vi "DiffDriveTrainSim_KitBotWheelSize.vi"(11 "Wheel Size":T1) -> (3 "WheelDiameter_M":dbl)   [LabVIEW 2019, in "Trajectory_Library.lvlib"]
doc: "Convience function to allow user to select kit bot wheels size from an enum selector and return the diameter in meters.\n\nInput:\n - Wheel Size -- Enumerated heel size selector\n\nOutput:\n - WheelDiameter_M -- Wheel diameter in meters."
uses:
  Trajectory_Library.lvlib
  Enum/DIFF_DRIVE_KitBot_WheelSize_ENUM.ctl
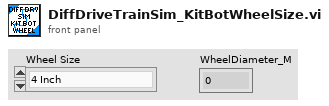
[diagram p1: front panel]
types:
  T1 = typedef "Trajectory_Library.lvlib/DIFF_DRIVE_KitBot_WheelSize_ENUM.ctl" = enum16{"4 Inch", "6 Inch", "8 Inch", "10 Inch"}
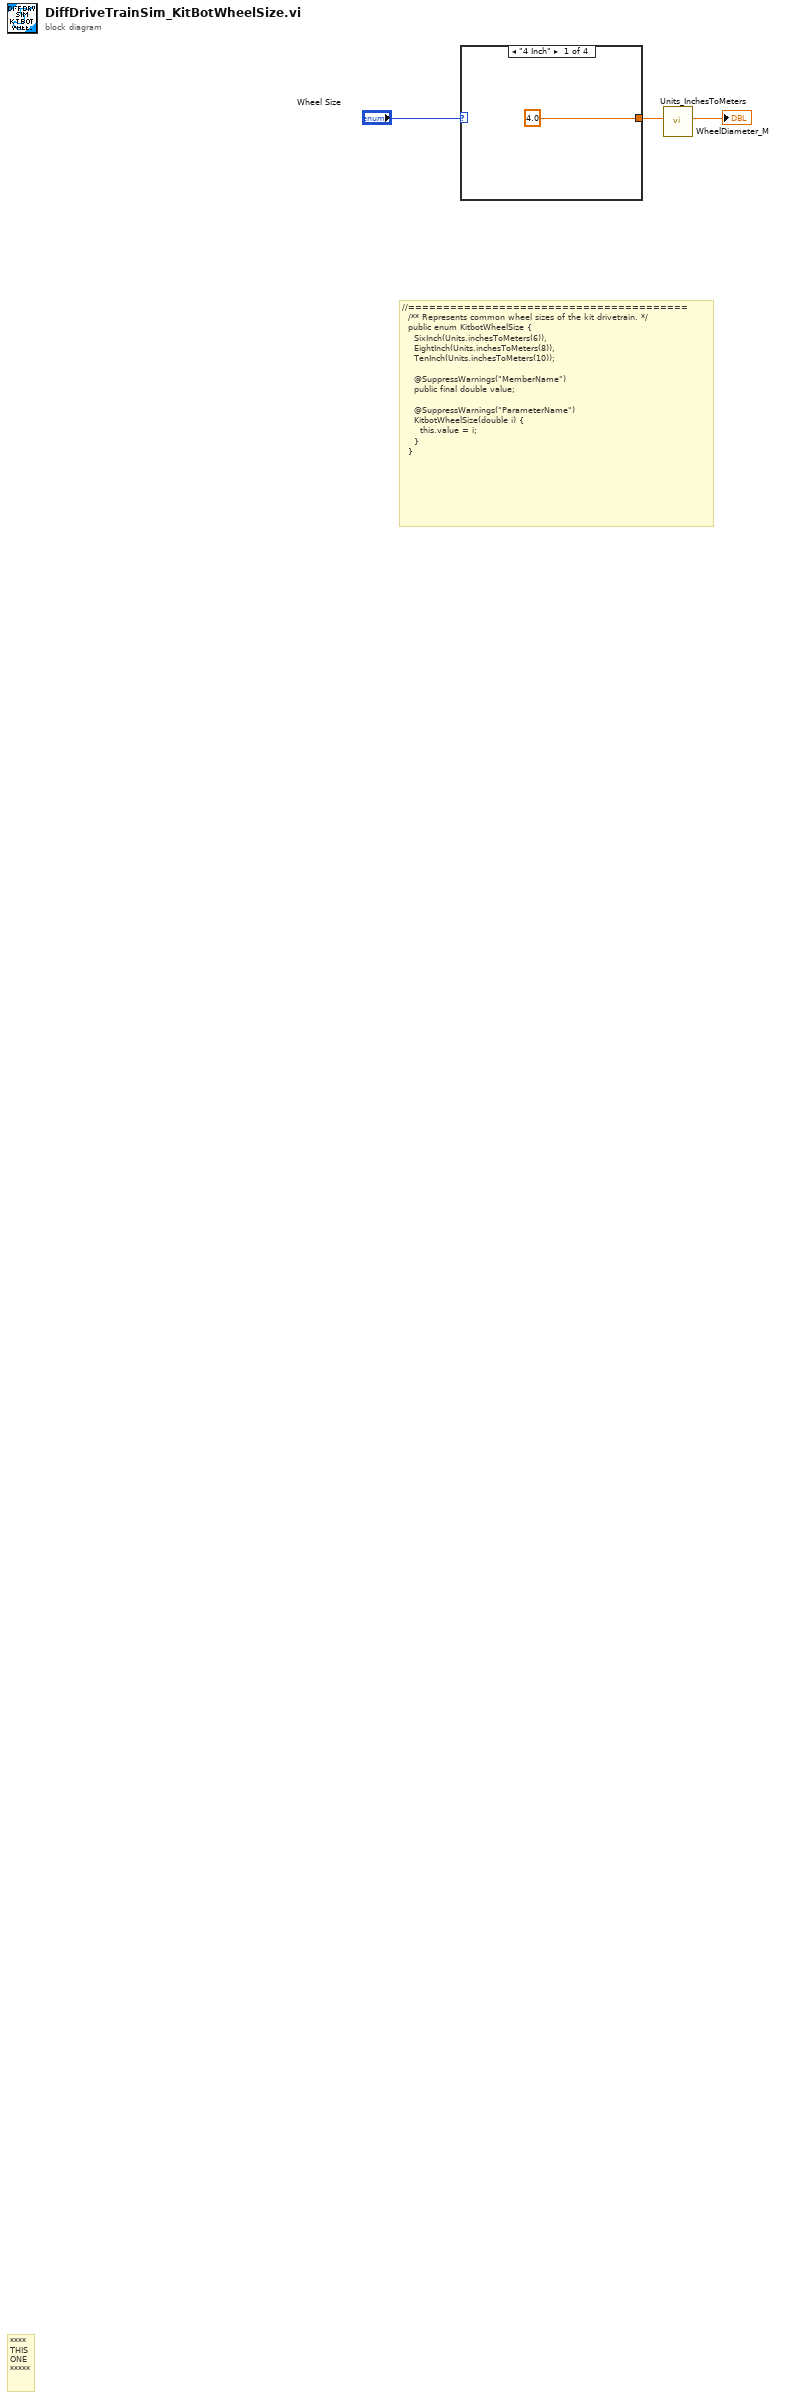
[diagram p0: block diagram]
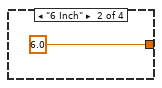
[diagram p2: hidden frame]
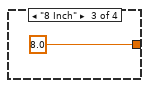
[diagram p3: hidden frame]
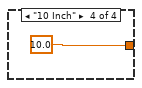
[diagram p4: hidden frame]
diagram:
  # "//========================================\n  /** Represents common wheel sizes of the kit drivetrain. */\n  public enum KitbotWheelSize {\n    SixInch(Units.inchesToMeters(6)),\n    EightInch(Units.inchesToMeters(8)),\n    TenInch(Units.inchesToMeters(10));\n\n    @SuppressWarnings(\"MemberName\")\n    public final double value;\n\n    @SuppressWarnings(\"ParameterName\")\n    KitbotWheelSize(double i) {\n      this.value = i;\n    }\n  }"
  # "****\nTHIS\nONE\n*****"
  n1 = case shown="\"4 Inch\"" "Wheel Size" {
    tunnel: [4.0 6.0 8.0 10.0] -> w2
    frame "4 Inch" {
    }
    frame "6 Inch" {
    }
    frame "8 Inch" {
    }
    frame "10 Inch" {
    }
  }
  n2 = call "Units_InchesToMeters.vi"("Inches"=w2) -> ("Meters"=→"WheelDiameter_M":dbl)  [unwired: 10 in]
